vi "NISE.remote.Read Dev.Properties.vi"(8 "error in (no error)":errorcluster, 11 "SLSC Remote in":refnum<class "SLSC Interface.lvclass">) -> (0 "error out":errorcluster, 2 "Dev.Properties":refnum<k21>[](array[refnum]), 3 "SLSC Remote out":refnum<class "SLSC Interface.lvclass">)   [LabVIEW 2016, in "SLSC Interface.lvclass"]
uses:
  SLSC Interface Class/SLSC Interface.lvclass
  <vilib>/NI/JSON Support for LabVIEW/JSON Value/Array/Index Array/Index Array (String).vi
  <vilib>/NI/JSON Support for LabVIEW/JSON Value/JSON Value.lvclass
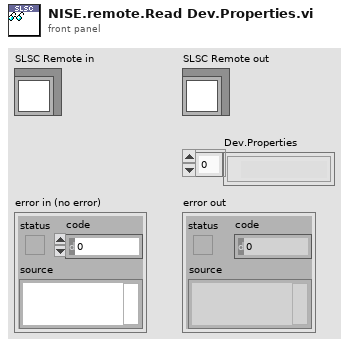
[diagram p1: front panel]
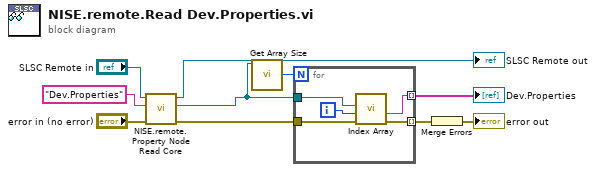
[diagram p0: block diagram]
diagram:
  n1 = call "NISE.remote.Property Node Read Core.vi"("error in (no error)"="error in (no error)", "property"="Dev.Properties", "SLSC Remote in"="SLSC Remote in") -> ("error out"=w6:errorcluster, "JSON Value out"=w1:refnum<class "JSON Value.lvclass">, "SLSC Remote out"=→"SLSC Remote out":refnum<class "SLSC Interface.lvclass">)  [unwired: 6 in]
  n2 = call <vilib>:"Get Array Size.vi"("JSON Value in"=w1) -> ("size(s)"=w5:i32)  [unwired: 9 in, 1 out]
  n3 = for {
    N: w5 -> [_]
    tunnel: w1 -> [w14]
    tunnel: w6 -> [w13]
    tunnel: [w12] -> w4 mode=indexing
    tunnel: [w11] -> w2 mode=indexing
    i -> [w15]
    n4 = call-poly <vilib>:"Index Array.vi"("error in (no error)"=w13, "index"=w15, "JSON Value in"=w14) -> ("error out"=w12:errorcluster, "String"=w11:string)  [unwired: 7 in]
  }
  "Dev.Properties" <- w2
  n5 = Merge Errors(w4) -> (→"error out":errorcluster)
